vi "Not.vi"(7 "Name":string="Not", 11 "Node In":refnum<class "abs_Node.lvclass">) -> (3 "Node":refnum<class "abs_Node.lvclass">)   [LabVIEW 2021, in "BT.lvlib"]
uses:
  BT.lvlib
  abs_Node/abs_Node.lvclass
  Not/Not.lvclass
  C:/Users/Tim/Documents/LabVIEW/2021/Behaviour Tree/abs_Decorator/abs_Decorator.lvclass
  C:/Users/Tim/Documents/LabVIEW/2021/Behaviour Tree/abs_Node/abs_Node.lvclass
  abs_Decorator/abs_Decorator.lvclass/abs_Decorator.ctl
  abs_Node/abs_Node.lvclass/abs_Node.ctl
  abs_Decorator/Properties/Write Node.vi
  abs_Node/Properties/Write Name.vi
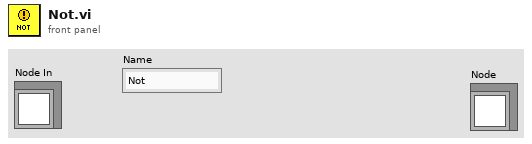
[diagram p1: front panel]
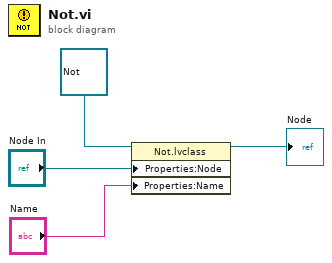
[diagram p0: block diagram]
diagram:
  n1 = property class="Not.lvclass"(reference=refnum<class "Not.lvclass"> refnum ("BT.lvlib:Not.lvclass"), "Properties:Node"="Node In", "Properties:Name"="Name") -> (reference out=→"Node":refnum<class "Not.lvclass">)  [unwired: 1 in, 1 out]
